vi "DeepLabv3_OpenVINO_imgs.vi"() -> ()   [LabVIEW 2018]
doc: "DeepLabv3_OpenVINO_imgs: This example is a semantic segmentation example of the DeepLabv3 model, which can be used for image semantic segmentation tasks. The ability to segment the input image into semantically meaningful regions and assign a semantic label to each pixel."
uses:
  vi.lib/VIRobotics/ModelZoo/Segmentation/Yiku_Seg_OpenVINO/Yiku_Seg_OpenVINO.lvclass
  vi.lib/VIRobotics/opencv_yiku/opencv_yiku.lvlib
panel:
  in  "device_name":string(combo)="CPU"
  in  "class_names_path":path=path "C:/ProgramData/VIRobotics/ModelZoo/Segmentation/class.txt"
  in  "model_file":path
  in  "stop":bool
  in  "imgs":i32(listbox)=1
  out "每帧耗时(s)":dbl
  out "picture":picture
  out "mask":picture
  in  "image Folder":path=path "C:/ProgramData/VIRobotics/ModelZoo/Segmentation/imgs"
  # "Overview: Demonstrates how to use OpenVINO to load the ONNX model of deeplabv3 for real-time image segmentation.\nRequirements: Windows.\nInstructions: \n1.Select the device_name to use.（If your computer has Intel GPU, you can select GPU in the \"type\" control before running the VI to achieve faster inference).\n2.Download the model of deeplabv3.Specify the model_file ,then run the VI.\n3.Click on the image in the imgs control on the right side of the interface that need to be detected.\nIf you want to load the model you trained, follow the following steps:\n1.Select the device_name to use. \n2.Specify the model_file and class_names_file.\n3.Run the VI.\n4.Specify the path of the image Folder and click on the image in the imgs control on the right side of the interface that need to be detected."
  # "Download the model of deeplabv3"
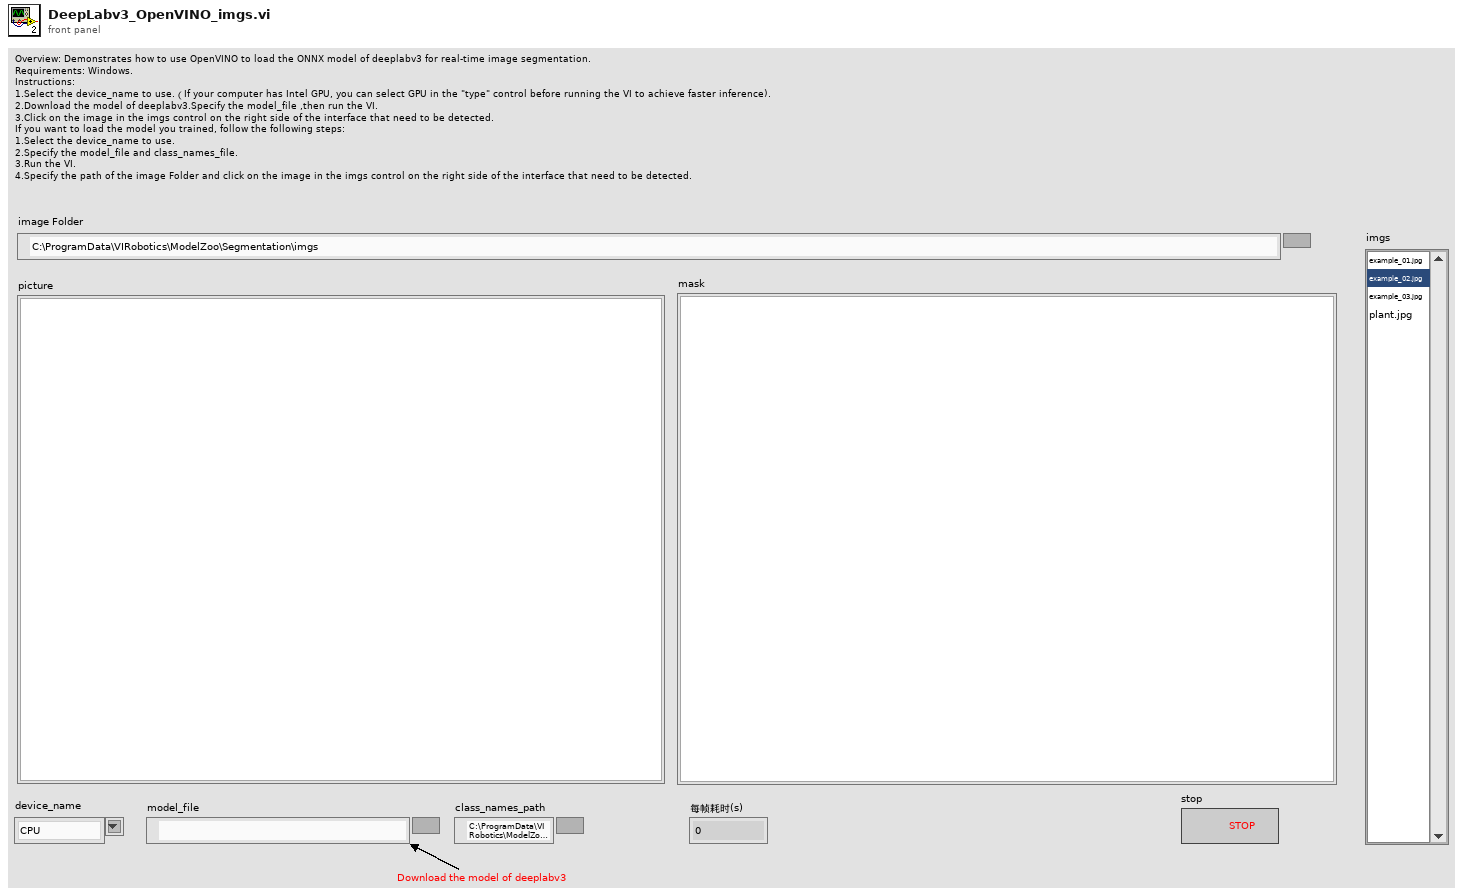
[diagram p1: front panel]
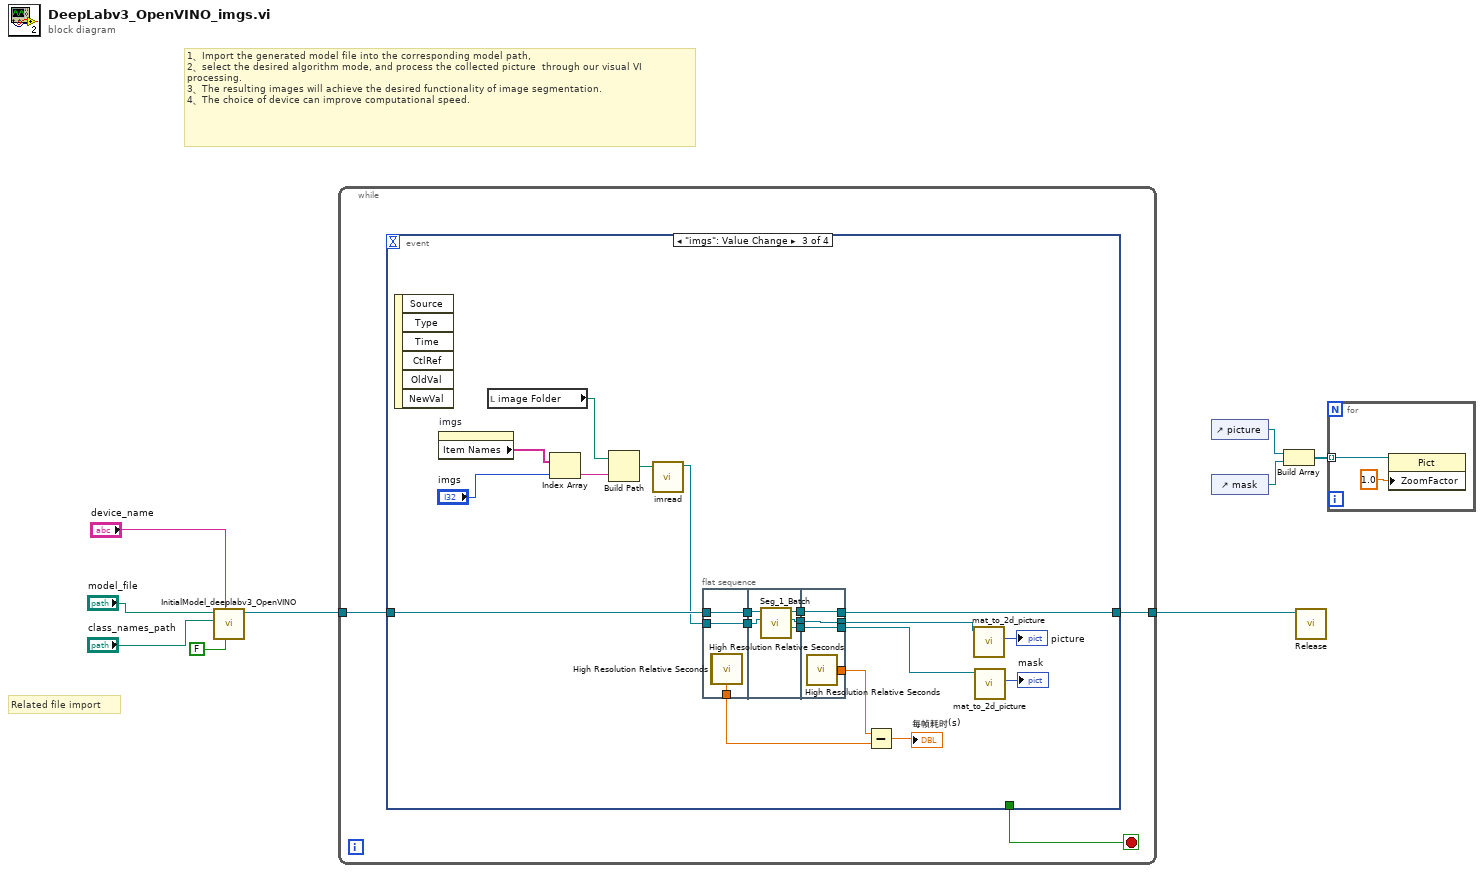
[diagram p0: block diagram]
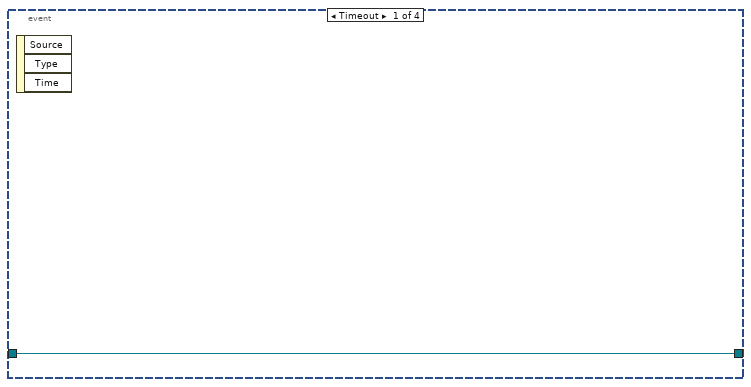
[diagram p2: hidden frame]
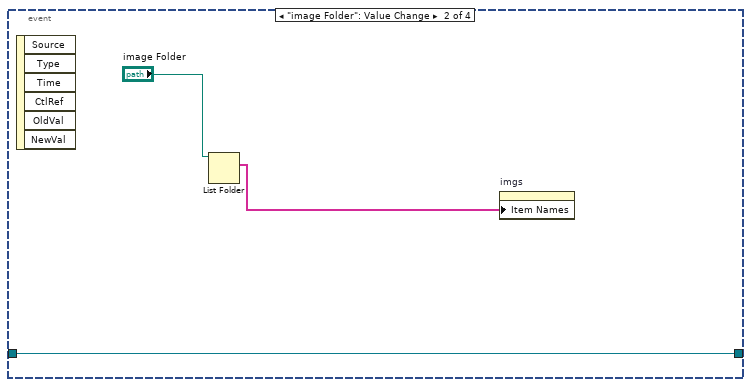
[diagram p3: hidden frame]
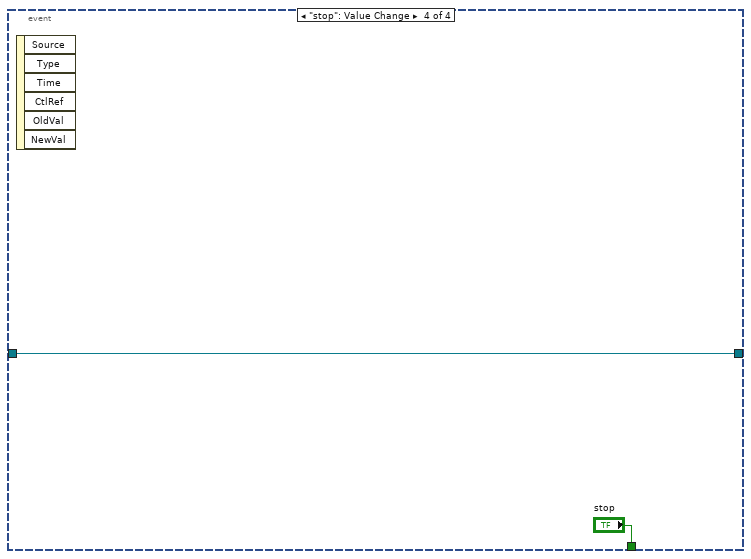
[diagram p4: hidden frame]
diagram:
  # "1、Import the generated model file into the corresponding model path, \n2、select the desired algorithm mode, and process the collected picture  through our visual VI processing. \n3、The resulting images will achieve the desired functionality of image segmentation. \n4、The choice of device can improve computational speed."
  # "Related file import"
  n1 = call "InitialModel_deeplabv3_OpenVINO.vi"("use letterbox"=FALSE, "device_name"="device_name", "class_names_path"="class_names_path", "path"="model_file") -> ("Seg_OV out"=w2:refnum<class "Yiku_Seg_OpenVINO.lvclass">)  [unwired: 6 in, 1 out]
  n2 = while {
    tunnel: w2 -> [w12]
    tunnel: [w11] -> w9
    stop <- w10 stop-if-true
    n3 = event shown="[2] \"imgs\": Value Change" {
      selector: _ -> [_ _ _ _]
      dyn-events: _ -> [_ _ _ _]
      timeout: _ -> [_ _ _ _]
      tunnel: w12 -> [w13 w14 w31 w49]
      tunnel: [w13 w14 w17 w49] -> w11
      tunnel: [_ _ _ "stop"] -> w10
      event Timeout {
        n4 = event-data() -> ()  [unwired: 1 in, 3 out]
      }
      event "image Folder": Value Change {
        n5 = event-data() -> ()  [unwired: 1 in, 6 out]
        n6 = List Folder(path="image Folder") -> (filenames=w15:string[])  [unwired: 3 in, 3 out]
        n7 = property on="imgs" class="LstBox (strict)"("Item Names"=w15) -> ()  [unwired: 2 in, 2 out]
      }
      event "imgs": Value Change {
        n8 = event-data() -> ()  [unwired: 1 in, 6 out]
        n9 = property on="imgs" class="LstBox (strict)"() -> ("Item Names"=w36:string[])  [unwired: 2 in, 2 out]
        n10 = local read "image Folder"() -> (w33:path)
        n11 = Index Array(array=w36, index="imgs") -> (element=w34:string)
        n12 = Build Path(base path=w33, name or relative path=w34) -> (appended path=w32:path)
        n13 = call "imread.vi"("path"=w32) -> ("Mat out"=w25:refnum<class "Mat_8U.lvclass">)  [unwired: 9 in, 1 out]
        n14 = flat-sequence {
          tunnel: w31 -> [w39]
          tunnel: [w39] -> w30
          tunnel: [w38] -> w27
          tunnel: w25 -> [w37]
          tunnel: [w37] -> w24
          tunnel: w30 -> [w44]
          tunnel: [w42] -> w29
          tunnel: w24 -> [w43]
          tunnel: [w41] -> w20
          tunnel: [w40] -> w18
          tunnel: [w48] -> w21
          tunnel: w29 -> [w48]
          tunnel: [w47] -> w28
          tunnel: w20 -> [w46]
          tunnel: [w46] -> w19
          tunnel: [w45] -> w17
          tunnel: w18 -> [w45]
          frame #0 {
            n15 = call <vilib>:"High Resolution Relative Seconds.vi"() -> ("relative seconds"=w38:dbl)
            n16 = call <vilib>:"High Resolution Relative Seconds.vi"() -> ()  [unwired: 1 out]
          }
          frame #1 {
            n17 = call-dynamic "Seg_1_Batch.vi"("img"=w43, "Seg_OV in"=w44) -> ("mask"=w41:refnum<class "Mat_8U.lvclass">, "img out"=w42:refnum<class "Mat_8U.lvclass">, "Seg_OV out"=w40:refnum<class "Yiku_Seg_OpenVINO.lvclass">)  [unwired: 6 in, 1 out]
          }
          frame #2 {
            n18 = call <vilib>:"High Resolution Relative Seconds.vi"() -> ("relative seconds"=w47:dbl)
          }
        }
        n19 = Subtract(x=w28, y=w27) -> (x-y=→"每帧耗时(s)":dbl)
        n20 = call "mat_to_2d_picture.vi"("Mat_8U in"=w21) -> ("picture"=→"picture":picture)  [unwired: 8 in, 2 out]
        n21 = call "mat_to_2d_picture.vi"("Mat_8U in"=w19) -> ("picture"=→"mask":picture)  [unwired: 8 in, 2 out]
      }
      event "stop": Value Change {
        n22 = event-data() -> ()  [unwired: 1 in, 6 out]
      }
    }
  }
  n23 = control-ref of="picture"() -> (w6:refnum<vi>)
  n24 = control-ref of="mask"() -> (w8:refnum<vi>)
  n25 = Build Array(w6, w8) -> (w7:refnum<vi>[])
  n26 = call-dynamic "Release.vi"("Seg_OV in"=w9) -> ()  [unwired: 9 in, 2 out]
  n27 = for {
    tunnel: w7 -> [w52] mode=indexing
    n28 = property class="Pict"(reference=w52, "ZoomFactor"=sgl 1.0 ("Zoom Factor")) -> ()  [unwired: 1 in, 2 out]
  }
